vi "Ball Kalman Filter And Update.vi"(10 "Cluster in":T4, 11 "Detection Ball":T1) -> (3 "Cluster out":T3)   [LabVIEW 2016]
uses:
  SSL Detection Ball.ctl
  <vilib>/Analysis/Matrix/Datatypes/RealMatrix.ctl
  Get Ball Pose.vi
  <vilib>/Analysis/Matrix/NI_Matrix.lvlib
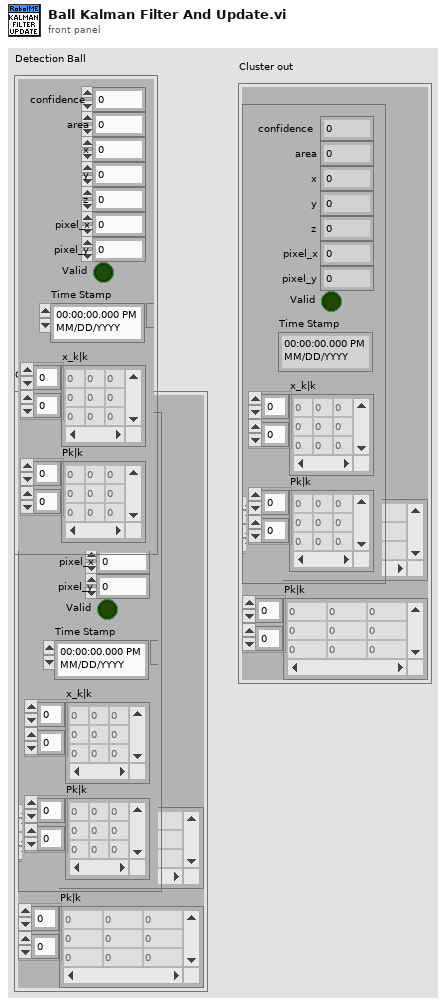
[diagram p1: front panel]
types:
  T1 = typedef "SSL Detection Ball.ctl" = cluster{"x":sgl, "area":u32, "confidence":sgl, "y":sgl, "z":sgl, "pixel_x":sgl, "pixel_y":sgl, "Valid":bool, "Time Stamp":timestamp, "x_k|k":T2, "Pk|k":T2}
  T2 = typedef "NI_Matrix.lvlib/RealMatrix.ctl" = dbl[][]
  T3 = cluster{"Detection Ball out":T1, "x_k|k":T2, "Pk|k":T2}
  T4 = cluster{"Detection Ball":T1, "Pose":T2, "Pk|k":T2}
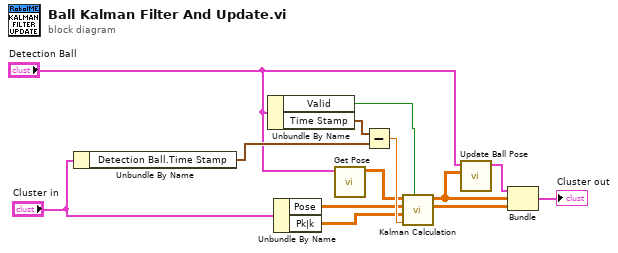
[diagram p0: block diagram]
diagram:
  n1 = Unbundle By Name("Cluster in") -> ("Detection Ball.Time Stamp"=w12:timestamp)
  n2 = Unbundle By Name("Detection Ball") -> ("Valid"=w9:bool, "Time Stamp"=w11:timestamp)
  n3 = Unbundle By Name("Cluster in") -> ("Pose"=w4:T2, "Pk|k"=w5:T2)
  n4 = call-poly "Get Pose.vi"("Detection Ball"="Detection Ball") -> ("Pose"=w1:T2)  [unwired: 10 in]
  n5 = Subtract(x=w11, y=w12) -> (x-y=w13:dbl)
  n6 = call "Kalman Calculation.vi"("Use Observation"=w9, "intervalo"=w13, "Pk-1|k-1"=w5, "x_k-1|k-1"=w4, "z_k"=w1) -> ("Pk|k"=w3:T2, "x_k|k"=w2:T2)  [unwired: 4 in, 1 out]
  n7 = call "Update Ball Pose.vi"("x_k|k"=w2, "Detection Ball in"="Detection Ball") -> ("Detection Ball out"=w7:T1)  [unwired: 9 in]
  n8 = Bundle("Detection Ball out"=w7, "x_k|k"=w2, "Pk|k"=w3) -> (→"Cluster out":T3)  [unwired: 1 in]
